vi "TEST3.vi"() -> ()   [LabVIEW 2015]
panel:
  out "x > 0?":bool
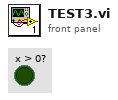
[diagram p1: front panel]
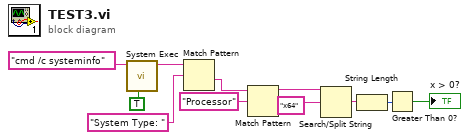
[diagram p0: block diagram]
diagram:
  n1 = call <vilib>:"System Exec.vi"("run minimized? (F)"=TRUE, "command line"="cmd /c systeminfo") -> ("standard output"=w9:string)  [unwired: 4 in, 5 out]
  n2 = Match Pattern(string=w9, regular expression="System Type: ") -> (after substring=w7:string)  [unwired: 1 in, 3 out]
  n3 = Match Pattern(string=w7, regular expression="Processor") -> (before substring=w5:string)  [unwired: 1 in, 3 out]
  n4 = Search/Split String(string=w5, search string/char (-)="x64" ("string")) -> (match + rest of string=w3:string)  [unwired: 1 in, 2 out]
  n5 = String Length(string=w3) -> (length=w2:i32)
  n6 = Greater Than 0?(x=w2) -> (x > 0?=→"x > 0?":bool)
